vi "Test Criteria, Mark Result Pass-Fail.vi"(6 "row (0)":i32, 8 "error in":errorcluster, 11 "Tbl Refnum":refnum<vi>) -> (0 "error out":errorcluster, 3 "Tbl Refnum out":refnum<vi>)   [LabVIEW 2010]
doc: "For Debug of the TesStand / LabView interface."
uses:
  Comparison Control.ctl
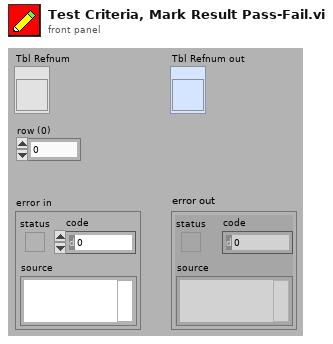
[diagram p1: front panel]
types:
  T1 = typedef "Comparison Control.ctl" = enum16{"EQ", "GE", "GELE", "GELT", "GT", "GTLE", "GTLT", "LE", "LT", "NE", "None"}
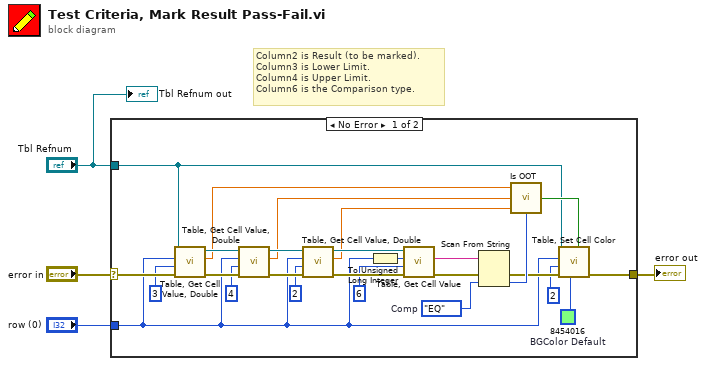
[diagram p0: block diagram]
diagram:
  # "Column2 is Result (to be marked).\nColumn3 is Lower Limit.\nColumn4 is Upper Limit.\nColumn6 is the Comparison type."
  n1 = case shown="No Error" "error in" {
    selector: "error in" -> [w30 w31]
    tunnel: [w10 w31] -> w4
    tunnel: "Tbl Refnum" -> [w8 _]
    tunnel: "row (0)" -> [w7 _]
    frame No Error {
      w6 = u32 8454016  # BGColor Default
      w16 = Comparison_Control."EQ"  # Comp
      n2 = call "Table, Get Cell Value, Double.vi"("error in"=w30, "col"=3 ("col_n"), "row"=w7, "Tbl Refnum"=w8) -> ("error out"=w25:errorcluster, "cell value"=w22:dbl, "Tbl Refnum out"=w28:refnum<vi>)  [unwired: 5 in]
      n3 = call "Table, Get Cell Value, Double.vi"("error in"=w25, "col"=4 ("col_n"), "row"=w7, "Tbl Refnum"=w28) -> ("error out"=w24:errorcluster, "cell value"=w21:dbl, "Tbl Refnum out"=w27:refnum<vi>)  [unwired: 5 in]
      n4 = call "Table, Get Cell Value, Double.vi"("error in"=w24, "col"=2 ("col_n"), "row"=w7, "Tbl Refnum"=w27) -> ("error out"=w23:errorcluster, "cell value"=w20:dbl, "Tbl Refnum out"=w26:refnum<vi>)  [unwired: 5 in]
      n5 = To Unsigned Long Integer(number=w7) -> (unsigned 32bit integer=w5:u32)
      n6 = call "Table, Get Cell Value.vi"("error in"=w23, "column (0)"=u32 6 ("col_n"), "row (0)"=w5, "Tbl Refnum"=w26) -> ("error out"=w15:errorcluster, "cell value"=w14:string)  [unwired: 5 in, 1 out]
      n7 = Scan From String(input string=w14, error in=w15, default 1=w16) -> (error out=w11:errorcluster, output 1=w13:T1)  [unwired: 2 in, 2 out]
      n8 = call "Is OOT.vi"("Comp"=w13, "Result"=w20, "UL"=w21, "LL"=w22) -> ("OOT"=w12:bool)
      n9 = call "Table, Set Cell Color.vi"("Enable (T)"=w12, "BGColor Default"=w6, "error in"=w11, "col (0)"=2, "row (0)"=w7, "Tbl Refnum"=w8) -> ("error out"=w10:errorcluster)  [unwired: 1 in, 3 out]
    }
    frame Error {
    }
  }
  "error out" <- w4
  "Tbl Refnum out" <- "Tbl Refnum"
